vi "Handle Command.vi"(8 "error in (no error)":errorcluster, 9 "Data":variant, 10 "Command":string, 11 "Sequence Experiment":refnum<class "Sequence Experiment.lvclass">) -> (0 "error out":errorcluster, 1 "Processed Data":variant, 2 "Command":string, 3 "Sequence Experiment out":refnum<class "Sequence Experiment.lvclass">)   [LabVIEW 2016, in "Sequence Experiment.lvclass"]
uses:
  Sequence Experiment.lvclass
  <userlib>/LevyLab/Levylab Instruments/SMOs/Instrument/Instrument.lvclass
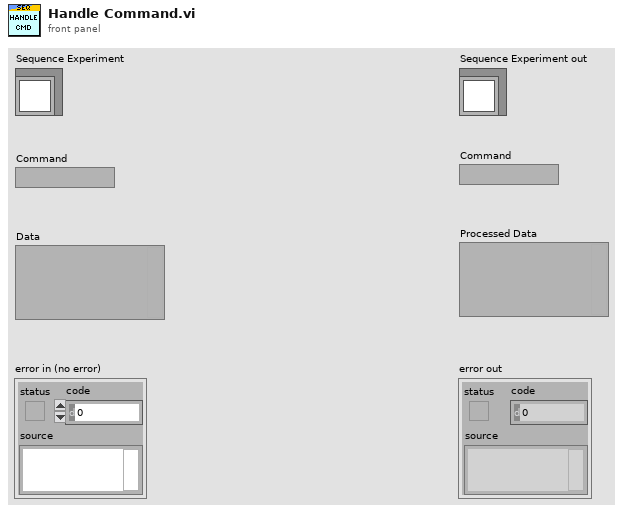
[diagram p1: front panel]
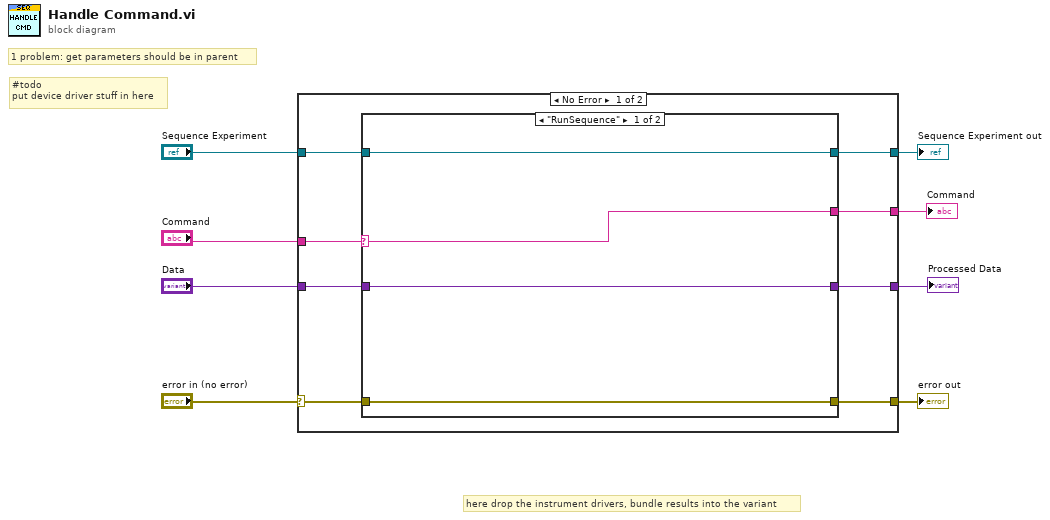
[diagram p0: block diagram]
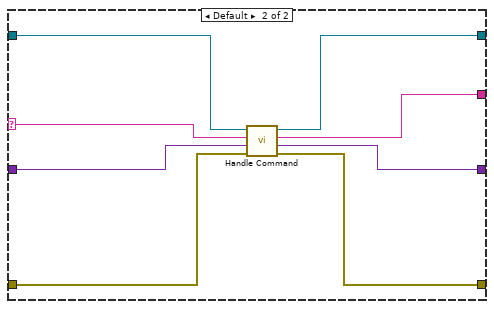
[diagram p2: hidden frame]
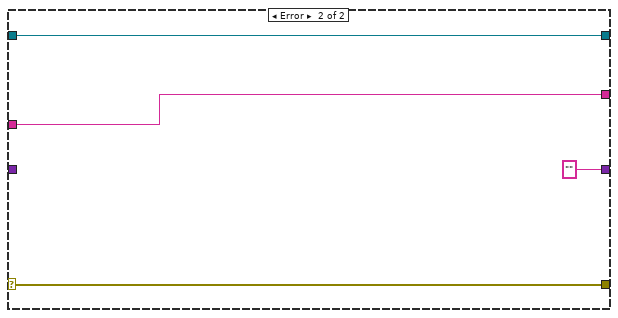
[diagram p3: hidden frame]
diagram:
  # "here drop the instrument drivers, bundle results into the variant"
  # "1 problem: get parameters should be in parent"
  # "#todo\nput device driver stuff in here"
  n1 = case shown="No Error" "error in (no error)" {
    selector: "error in (no error)" -> [w12 w32]
    tunnel: [w10 w32] -> w6
    tunnel: [w14 w31] -> w5
    tunnel: "Sequence Experiment" -> [w15 w31]
    tunnel: "Command" -> [w16 w29]
    tunnel: [w13 "" ("String")] -> w3
    tunnel: "Data" -> [w11 _]
    tunnel: [w9 w29] -> w1
    frame No Error {
      n2 = case shown="\"RunSequence\"" w16 {
        selector: w16 -> [w20 w28]
        tunnel: w15 -> [w19 w25]
        tunnel: [w19 w22] -> w14
        tunnel: [w18 w24] -> w13
        tunnel: w12 -> [w17 w26]
        tunnel: w11 -> [w18 w27]
        tunnel: [w17 w23] -> w10
        tunnel: [w20 w21] -> w9
        frame "RunSequence" {
        }
        frame Default {
          n3 = call-parent "Handle Command.vi"("error in (no error)"=w26, "Data"=w27, "Command"=w28, "Instrument in"=w25) -> ("error out"=w23:errorcluster, "Processed Data"=w24:variant, "Command"=w21:string, "Instrument out"=w22:refnum<class "Sequence Experiment.lvclass">)  [unwired: 4 in]
        }
      }
    }
    frame Error {
    }
  }
  "error out" <- w6
  "Sequence Experiment out" <- w5
  "Command" <- w1
  "Processed Data" <- w3
